vi "Coord window-Idle case logic.vi"() -> (1 "Stop application":bool, 3 "Coordinates":cluster{"X":sgl, "Y":sgl, "Z":sgl})   [LabVIEW 2013]
uses:
  Global Variables/General Globals.vi
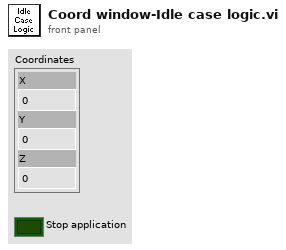
[diagram p1: front panel]
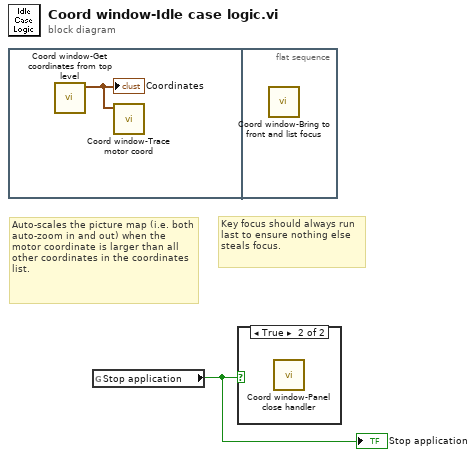
[diagram p0: block diagram]
diagram:
  # "Auto-scales the picture map (i.e. both auto-zoom in and out) when the motor coordinate is larger than all other coordinates in the coordinates list."
  # "Key focus should always run last to ensure nothing else steals focus."
  n1 = flat-sequence {
    frame #0 {
      n2 = call "Coord window-Get coordinates from top level.vi"() -> ("Coordinates"=w2:cluster{"X":sgl, "Y":sgl, "Z":sgl})  [unwired: 11 in]
      "Coordinates" <- w2
      n3 = call "Coord window-Trace motor coord.vi"("Coordinates"=w2) -> ()  [unwired: 11 in]
    }
    frame #1 {
      n4 = call "Coord window-Bring to front and list focus.vi"() -> ()  [unwired: 12 in]
    }
  }
  n5 = global read "General Globals.vi" "Stop application"() -> (w1:bool)
  "Stop application" <- w1
  n6 = case shown="True" w1 {
    frame False {
    }
    frame True {
      n7 = call "Coord window-Panel close handler.vi"() -> ()  [unwired: 12 in]
    }
  }
